vi "Get Result.vi"(6 "Last request":bool, 8 "error in (no error)":errorcluster, 11 "Instrument Recorder in":refnum<class "Pulse Recorder.lvclass">) -> (0 "error out":errorcluster, 2 "Result":refnum<class "Acquired Result.lvclass">, 3 "Instrument Recorder out":refnum<class "Pulse Recorder.lvclass">)   [LabVIEW 2018, in "Pulse Recorder.lvclass"]
uses:
  Pulse Recorder.lvclass
  NHMFL_Core/Libraries/Instruments/Results/Acquired Result/Acquired Result.lvclass
  NHMFL_Core/Libraries/Instruments/Results/Acquired Result/Acquired Result.lvclass/Acquired Result.ctl
  NHMFL_Core/Libraries/Instruments/Results/Acquired Result/Read Final.vi
  Instrument Actor/Instrument Actor.lvclass
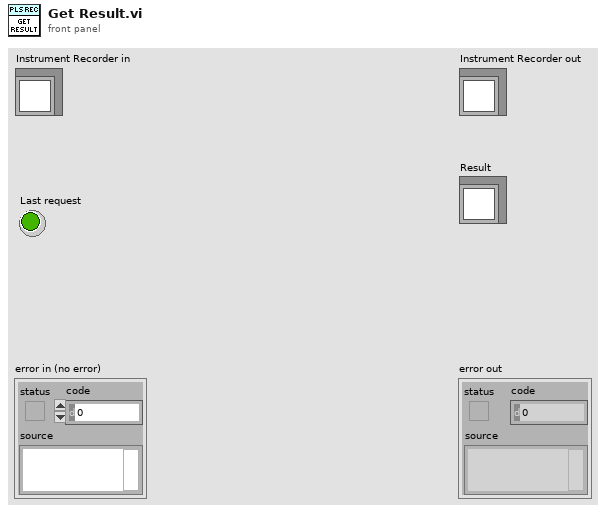
[diagram p1: front panel]
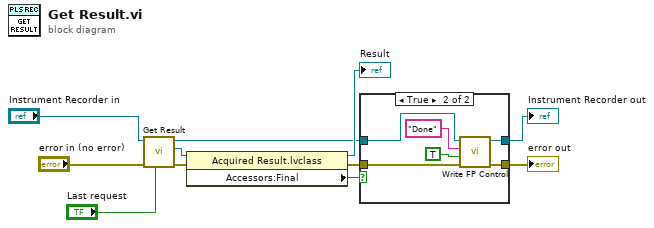
[diagram p0: block diagram]
diagram:
  n1 = call-parent "Get Result.vi"("Last request"="Last request", "error in (no error)"="error in (no error)", "Instrument Recorder in"="Instrument Recorder in") -> ("error out"=w11:errorcluster, "Result"=w7:refnum<class "Acquired Result.lvclass">, "Instrument Recorder out"=w1:refnum<class "Pulse Recorder.lvclass">)  [unwired: 6 in]
  n2 = property class="Acquired Result.lvclass"(reference=w7, error in=w11) -> (reference out=→"Result":refnum<class "Acquired Result.lvclass">, error out=w4:errorcluster, "Accessors:Final"=w5:bool)
  n3 = case shown="True" w5 {
    tunnel: w4 -> [w13 w17]
    tunnel: [w13 w16] -> w3
    tunnel: [w12 w15] -> w2
    tunnel: w1 -> [w12 w14]
    frame False {
    }
    frame True {
      n4 = call-dynamic "Write FP Control.vi"("error in (no error)"=w17, "Control Value"=TRUE, "Control Name"="Done", "Measure Object in"=w14) -> ("error out"=w16:errorcluster, "Measure Object out"=w15:refnum<class "Pulse Recorder.lvclass">)  [unwired: 6 in]
    }
  }
  "error out" <- w3
  "Instrument Recorder out" <- w2
